vi "MainScript.vi"() -> ()   [LabVIEW 2020]
uses:
  <vilib>/Platform/TimedLoop/XDataNode/timing_clust.ctl
  <vilib>/Platform/TimedLoop/XDataNode/nitl_modes.ctl
  <vilib>/Platform/TimedLoop/XDataNode/wakeup.ctl
  Global 2.vi
  <vilib>/imath/engines/lvmath2/RunTimeEngine/Managers/WorkSpace/UID Generator.vi
  <vilib>/imath/engines/lvmath2/RunTimeEngine/RunTimeType/NIMS_RunTimeType_From StrictType (excl LVString).vi
  <instcachedir>/0/NIMS_RunTimeType_From StrictType (excl LVString)_283B1B2000484AAA8744D21CE97EA49F.lvgen/NIMS_RunTimeType_From StrictType (excl LVString)_283B1B2000484AAA8744D21CE97EA49F_000.vi
  <vilib>/imath/engines/lvmath2/RunTimeEngine/LocalVariableDefStatement/MC_LocalVariableDefStatement_Display.vi
  <vilib>/imath/engines/lvmath2/RunTimeEngine/Managers/SymbolTable/Clear UID.vi
  <vilib>/imath/engines/lvmath2/RunTimeEngine/NodeEndStatement/NIMS_NodeEndStatement_Output.vi
  <instcachedir>/0/NIMS_NodeEndStatement_Output_53EC0D466D134D7ABD903AC30B43404B.lvgen/NIMS_NodeEndStatement_Output_53EC0D466D134D7ABD903AC30B43404B_005.vi
  <vilib>/imath/engines/lvmath2/RunTimeEngine/ErrorHandling/NIMS_Finalize Error.vi
  <vilib>/Platform/TimedLoop/XDataNode/loadnilvce.vi
  <vilib>/imath/engines/lvmath2/RunTimeEngine/RangeToken/NIMS_Range_R2 - Integer.vi
  <instcachedir>/0/NIMS_Range_R2 - Integer_FFC1A4B1B9F04947ABCB56F009996D55.lvgen/NIMS_Range_R2 - Integer_FFC1A4B1B9F04947ABCB56F009996D55_000.vi
  <vilib>/imath/engines/lvmath2/RunTimeEngine/CommandStatement/MC_CommandStatement_break.vi
  <vilib>/imath/engines/lvmath2/RunTimeEngine/MatrixToken/NIMS_MatrixToken_M_SorCV.vi
  <instcachedir>/0/NIMS_MatrixToken_M_SorCV_D62667310BD447638EB690CBF8A818C2.lvgen/NIMS_MatrixToken_M_SorCV_D62667310BD447638EB690CBF8A818C2_000.vi
  <vilib>/imathl/engines/lvmath/Functions/Error Handling/Create Error.vi
  <vilib>/imath/engines/lvmath2/RunTimeEngine/IndexRead/NIMS M(S).vi
  <instcachedir>/0/NIMS M(S)_B826C018497E4940AE96BD27B540B6FB.lvgen/NIMS M(S)_B826C018497E4940AE96BD27B540B6FB_000.vi
  <vilib>/imath/engines/lvmath2/RunTimeEngine/MatrixToken/NIMS_MatrixToken_M_M.vi
  <instcachedir>/0/NIMS_MatrixToken_M_M_70A974A5272043BBA0045176BCC4D8A7.lvgen/NIMS_MatrixToken_M_M_70A974A5272043BBA0045176BCC4D8A7_004.vi
  <vilib>/imath/engines/lvmath2/RunTimeEngine/ErrorHandling/NIMS_Create Error From Enums.vi
  <vilib>/imath/engines/lvmath2/RunTimeEngine/BuiltInFunctions/length/NIMS_length(GV).vi
  <instcachedir>/0/NIMS_length(GV)_08A3D13377FD4E4B96F5795FBF3698FA.lvgen/NIMS_length(GV)_08A3D13377FD4E4B96F5795FBF3698FA_000.vi
  <vilib>/imath/engines/lvmath2/RunTimeEngine/BuiltInFunctions/zeros/NIMS_V=zeros(I32,I32).vi
  <vilib>/imath/engines/lvmath2/RunTimeEngine/RowToken/NIMS_RowToken_CV_CV.vi
  <instcachedir>/0/NIMS_RowToken_CV_CV_E2834F2F68C5494A92C49C498959A73E.lvgen/NIMS_RowToken_CV_CV_E2834F2F68C5494A92C49C498959A73E_000.vi
  <vilib>/imath/engines/lvmath2/RunTimeEngine/RowToken/NIMS_RowToken_M_CV.vi
  <instcachedir>/0/NIMS_RowToken_M_CV_79C297319A314039B767729C6880A213.lvgen/NIMS_RowToken_M_CV_79C297319A314039B767729C6880A213_000.vi
  <vilib>/imath/engines/lvmath2/RunTimeEngine/BuiltInFunctions/size/NIMS_[I32,I32]=size(GM).vi
  <instcachedir>/0/NIMS_[I32,I32]=size(GM)_B0A6EC1255BB4C8AB801FE6F734128D9.lvgen/NIMS_[I32,I32]=size(GM)_B0A6EC1255BB4C8AB801FE6F734128D9_000.vi
  <vilib>/imath/engines/lvmath2/RunTimeEngine/IndexRead/NIMS M($,S).vi
  <instcachedir>/0/NIMS M($,S)_3E5749BBB62E49528D4765A77F1F6D98.lvgen/NIMS M($,S)_3E5749BBB62E49528D4765A77F1F6D98_000.vi
  <vilib>/imath/engines/lvmath2/RunTimeEngine/ArithmeticOperatorToken/NIMS_ArithmeticOperator_plus.vi
  <instcachedir>/0/NIMS_ArithmeticOperator_plus_54468E2FAC2848C4BF0D457641184E60.lvgen/NIMS_ArithmeticOperator_plus_54468E2FAC2848C4BF0D457641184E60_004.vi
  <vilib>/imath/engines/lvmath2/RunTimeEngine/IndexRead/NIMS M(S,$).vi
  <instcachedir>/0/NIMS M(S,$)_F24F360562DE41D8BE234322A2E15C65.lvgen/NIMS M(S,$)_F24F360562DE41D8BE234322A2E15C65_000.vi
  <instcachedir>/0/NIMS_NodeEndStatement_Output_53EC0D466D134D7ABD903AC30B43404B.lvgen/NIMS_NodeEndStatement_Output_53EC0D466D134D7ABD903AC30B43404B_002.vi
  <vilib>/imath/engines/lvmath2/RunTimeEngine/IndexReplace/NIMS M(S,S)=S.vi
  <instcachedir>/0/NIMS M(S,S)=S_FBAB070788A64735BCFA47F7F92815DB.lvgen/NIMS M(S,S)=S_FBAB070788A64735BCFA47F7F92815DB_000.vi
  <instcachedir>/0/NIMS M(S,S)=S_FBAB070788A64735BCFA47F7F92815DB.lvgen/NIMS M(S,S)=S_FBAB070788A64735BCFA47F7F92815DB_002.vi
  <vilib>/imath/engines/lvmath2/RunTimeEngine/CommandStatement/NIMS_CommandStatement_MaskErr.vi
  <vilib>/imath/engines/lvmath2/RunTimeEngine/ArithmeticOperatorToken/NIMS_ArithmeticOperator_multmx-internal.vi
  <instcachedir>/0/NIMS_ArithmeticOperator_multmx-internal_B44B9A6937C8407A9A8862E3F2935EB3.lvgen/NIMS_ArithmeticOperator_multmx-internal_B44B9A6937C8407A9A8862E3F2935EB3_004.vi
  <vilib>/imath/engines/lvmath2/RunTimeEngine/BuiltInFunctions/length/NIMS_length(GM).vi
  <instcachedir>/0/NIMS_length(GM)_47CEC356FCE0482D9BA47DC61C99F2C7.lvgen/NIMS_length(GM)_47CEC356FCE0482D9BA47DC61C99F2C7_000.vi
  <instcachedir>/0/NIMS M(S)_B826C018497E4940AE96BD27B540B6FB.lvgen/NIMS M(S)_B826C018497E4940AE96BD27B540B6FB_005.vi
  <vilib>/imath/engines/lvmath2/RunTimeEngine/ArithmeticOperatorToken/NIMS_ArithmeticOperator_multmx(M,CV)-internal.vi
  <instcachedir>/0/NIMS_ArithmeticOperator_multmx(M,CV)-internal_19A14CC5BE0A4D31BE1E94A2E998D8C3.lvgen/NIMS_ArithmeticOperator_multmx(M,CV)-internal_19A14CC5BE0A4D31BE1E94A2E998D8C3_001.vi
  <vilib>/imath/engines/lvmath2/RunTimeEngine/IndexReplace/NIMS M($,S)=V.vi
  <instcachedir>/0/NIMS M($,S)=V_85A28EB895514E96A13A10261726EE3A.lvgen/NIMS M($,S)=V_85A28EB895514E96A13A10261726EE3A_001.vi
  <vilib>/imath/engines/lvmath2/RunTimeEngine/RowToken/NIMS_RowToken_M_M.vi
  <instcachedir>/0/NIMS_RowToken_M_M_23B851CD98934479877138710C79658F.lvgen/NIMS_RowToken_M_M_23B851CD98934479877138710C79658F_004.vi
  <vilib>/imath/engines/lvmath2/RunTimeEngine/IndexReplace/NIMS M(S)=S.vi
  <instcachedir>/0/NIMS M(S)=S_033E230F5F1E47BAA81748F03F1A64B6.lvgen/NIMS M(S)=S_033E230F5F1E47BAA81748F03F1A64B6_001.vi
  <vilib>/imath/engines/lvmath2/RunTimeEngine/NodeEndStatement/NIMS_NodeEndStatement_Get Vector.vi
  <instcachedir>/0/NIMS_NodeEndStatement_Get Vector_F9EEA26507564AFBA1E30D500A99934B.lvgen/NIMS_NodeEndStatement_Get Vector_F9EEA26507564AFBA1E30D500A99934B_001.vi
  <vilib>/imath/engines/lvmath/Functions/Error Handling/MergeErrorsWrapper.vi
  <instcachedir>/0/NIMS_NodeEndStatement_Output_53EC0D466D134D7ABD903AC30B43404B.lvgen/NIMS_NodeEndStatement_Output_53EC0D466D134D7ABD903AC30B43404B_009.vi
  <vilib>/imath/engines/lvmath2/RunTimeEngine/BuiltInFunctions/norm/NIMS_norm(GV,DBL).vi
  <instcachedir>/0/NIMS_norm(GV,DBL)_118B4CCB667A4D7498CD7C123070720C.lvgen/NIMS_norm(GV,DBL)_118B4CCB667A4D7498CD7C123070720C_000.vi
  <vilib>/imath/engines/lvmath2/RunTimeEngine/IndexRead/NIMS V(S).vi
  <instcachedir>/0/NIMS V(S)_0488751826AF41519A22953C041130DC.lvgen/NIMS V(S)_0488751826AF41519A22953C041130DC_000.vi
  <vilib>/imath/engines/lvmath2/RunTimeEngine/BuiltInFunctions/abs/NIMS_abs(signed).vi
  <instcachedir>/0/NIMS_abs(signed)_C4FCB8E6058B49B797C7C8D53CA5F6EC.lvgen/NIMS_abs(signed)_C4FCB8E6058B49B797C7C8D53CA5F6EC_000.vi
  <instcachedir>/0/NIMS_NodeEndStatement_Output_53EC0D466D134D7ABD903AC30B43404B.lvgen/NIMS_NodeEndStatement_Output_53EC0D466D134D7ABD903AC30B43404B_001.vi
  <vilib>/imath/engines/lvmath2/RunTimeEngine/BuiltInFunctions/cos/NIMS_cos(C).vi
  <instcachedir>/0/NIMS_cos(C)_9DC0D0878EF24EB8B280F2BED1FF8FCD.lvgen/NIMS_cos(C)_9DC0D0878EF24EB8B280F2BED1FF8FCD_001.vi
  <vilib>/imath/engines/lvmath2/RunTimeEngine/BuiltInFunctions/acos/NIMS_acos(C).vi
  <instcachedir>/0/NIMS_acos(C)_5BB0E87CCFB0408A9DC8B350AC83525E.lvgen/NIMS_acos(C)_5BB0E87CCFB0408A9DC8B350AC83525E_001.vi
  <instcachedir>/0/NIMS_RunTimeType_From StrictType (excl LVString)_283B1B2000484AAA8744D21CE97EA49F.lvgen/NIMS_RunTimeType_From StrictType (excl LVString)_283B1B2000484AAA8744D21CE97EA49F_009.vi
  <instcachedir>/0/NIMS_abs(signed)_C4FCB8E6058B49B797C7C8D53CA5F6EC.lvgen/NIMS_abs(signed)_C4FCB8E6058B49B797C7C8D53CA5F6EC_002.vi
  <vilib>/imath/engines/lvmath2/RunTimeEngine/RunTimeType/NIMS_RunTimeType_Set Source Original Bool.vi
  <instcachedir>/0/NIMS_NodeEndStatement_Output_53EC0D466D134D7ABD903AC30B43404B.lvgen/NIMS_NodeEndStatement_Output_53EC0D466D134D7ABD903AC30B43404B_010.vi
  <vilib>/platform/TimedLoop/XDataNode/XDataNode.xnode
  <vilib>/Platform/TimedLoop/XDataNode/XDNodeRunTimeDep.lvlib
  <vilib>/imath/engines/lvmath2/RunTimeEngine/Managers/SymbolTable/NIMS_WorkSpace.lvlib
panel:
  out "v2":dbl(graph)=-75141.23523042882
  out "v1":dbl(graph)=57052.989399066195
  out "Boolean":bool
  in  "CDB":dbl=-0.002
  in  "ThrustCoefB":dbl=0.00015
  in  "KdB":dbl
  in  "KiB":dbl
  in  "KpB":dbl=5.0
  in  "Reverse":bool
  out "Array":dbl[](array[numeric])=[-97.53326262976505, 22.07402728985534, 0.0]
  in  "CD":dbl=-0.002
  in  "Radio Buttons":enum32{"Racetrack", "Circular", "Tube"}(radio)=enum."Circular"
  in  "Racetrack length [mm]":dbl=60.0
  in  "Ractrack width [mm]":dbl=15.0
  out "Rotation speed [Hz]":dbl(graph)=50.0
  in  "Zscale":dbl=0.95
  in  "YScale":dbl=0.9
  in  "XScale":dbl=0.95
  in  "Zoffset":dbl=-0.073
  in  "Yoffset":dbl=-0.076
  in  "Xoffset":dbl=0.07
  out "?":bool
  in  "Centripedal force compensation":bool
  in  "KCentripedal force":dbl=0.007
  in  "?":bool=TRUE
  in  "Rot [Hz]":dbl=50.0
  in  "Rotational speed":bool
  in  "Traj_Rotate":bool
  in  "Omega_Max_change":dbl=20.0
  in  "Thrust coefficient [N.s/rad]":dbl=0.0002
  out "T4":dbl=29.408844544558946
  out "T1":dbl=27.525528387426544
  out "T2":dbl=30.561149827671912
  out "T3":dbl=31.865396803696214
  out "T5":dbl=28.858824483224712
  out "T6":dbl=28.760553201657874
  out "Z-":dbl(slide)=27.525528387426544 scale=0.0..100.0
  out "Z+":dbl(slide)=30.561149827671912 scale=0.0..100.0
  out "X-":dbl(slide)=31.865396803696214 scale=0.0..100.0
  out "X+":dbl(slide)=29.408844544558946 scale=0.0..100.0
  out "Y-":dbl(slide)=28.858824483224712 scale=0.0..100.0
  out "Y+":dbl(slide)=28.760553201657874 scale=0.0..100.0
  out "OverTemp":bool
  in  "Max Temp[C]":dbl=75.0
  in  "On Off":bool
  in  "Max Orientation change rate [rad/s]":dbl=15.0
  out "On":bool
  in  "Reset Integral":bool
  in  "Force Vertical":bool
  in  "Robot Mass [Kg]":dbl=5e-05
  in  "Kd":dbl
  in  "Ki":dbl=1e-05
  in  "Kp":dbl=0.5
  out "XZ View":T1(graph)=[{"XCircleBot"=[0.0114245818886292, 0.011179747012409945, 0.010505186500365478, 0.009566056291964605, 0.008592288215534915, 0.007822294657535332, 0.007444596895428308, 0.007551668514047607, 0.008117294646901975, 0.00900299028976764, 0.009991906259555651, 0.010841921437211719, 0.011344922461929932], "YCircleBot"=[-0.07472721060762046, -0.07376835953041205, -0.07304426863800466, -0.07273222063441234, -0.07290861575396909, -0.07353026631941255, -0.07444497059150072, -0.07542877706299969, -0.07624081559823631, -0.07668227084295065, -0.07664505915694673, -0.07613829125876125, -0.0752860416040183]}, {"XCircleBot"=array[1002 elements], "YCircleBot"=array[1002 elements]}, {"XCircleBot"=[0.008713695894261728, 0.008468861018042473, 0.007794300505998007, 0.006855170297597133, 0.005881402221167443, 0.0051114086631678605, 0.0047337109010608365, 0.004840782519680135, 0.0054064086525345036, 0.0062921042954001685, 0.0072810202651881805, 0.008131035442844247, 0.008634036467562459], "YCircleBot"=[0.0, 0.000958851077208406, 0.0016829419696157931, 0.001994989973208109, 0.0018185948536513636, 0.0011969442882079132, 0.0002822400161197344, -0.0007015664553792397, -0.0015136049906158565, -0.001955060235330194, -0.001917848549326277, -0.001411080651140784, -0.0005588309963978518]}, {"XCircleBot"=[0.0094245818886292, 0.012626616728347043], "YCircleBot"=[-0.07472721060762046, -0.02564219522787055]}]
  out "XY View":T1(graph)=[{"XCircleBot"=[0.0114245818886292, 0.011179747012409945, 0.010505186500365478, 0.009566056291964605, 0.008592288215534915, 0.007822294657535332, 0.007444596895428308, 0.007551668514047607, 0.008117294646901975, 0.00900299028976764, 0.009991906259555651, 0.010841921437211719, 0.011344922461929932], "YCircleBot"=[0.041338273099899805, 0.04229712417710821, 0.043021215069515596, 0.04333326307310791, 0.04315686795355117, 0.04253521738810772, 0.04162051311601954, 0.040636706644520564, 0.03982466810928395, 0.03938321286456961, 0.03942042455057353, 0.03992719244875902, 0.040779442103501956]}, {"XCircleBot"=array[1002 elements], "YCircleBot"=array[1002 elements]}, {"XCircleBot"=[0.008713695894261728, 0.008468861018042473, 0.007794300505998007, 0.006855170297597133, 0.005881402221167443, 0.0051114086631678605, 0.0047337109010608365, 0.004840782519680135, 0.0054064086525345036, 0.0062921042954001685, 0.0072810202651881805, 0.008131035442844247, 0.008634036467562459], "YCircleBot"=[0.029239122486290382, 0.03019797356349879, 0.030922064455906176, 0.031234112459498493, 0.031057717339941747, 0.030436066774498297, 0.029521362502410116, 0.028537556030911144, 0.027725517495674527, 0.027284062250960188, 0.027321273936964104, 0.0278280418351496, 0.02868029148989253]}, {"XCircleBot"=[0.0094245818886292, 0.012626616728347043], "YCircleBot"=[0.041338273099899805, 0.03237120902881452]}]
  out "Loop Duration [ms]":u32(graph)=3
  out "Max Current [A]":dbl(knob)=3.0 scale=0.0..2.0
  out "Current Saturation":bool=TRUE
  in  "Max Current [A]":dbl=3.0
  in  "Flux density magnitude (mT)":dbl=3.0
  in  "stop":bool
  # "Program performance monitoring"
  # "Program control"
  # "User Input"
  # "Auto"
  # "Manual"
  # "Show Direction Setpoint"
  # "Current control mode"
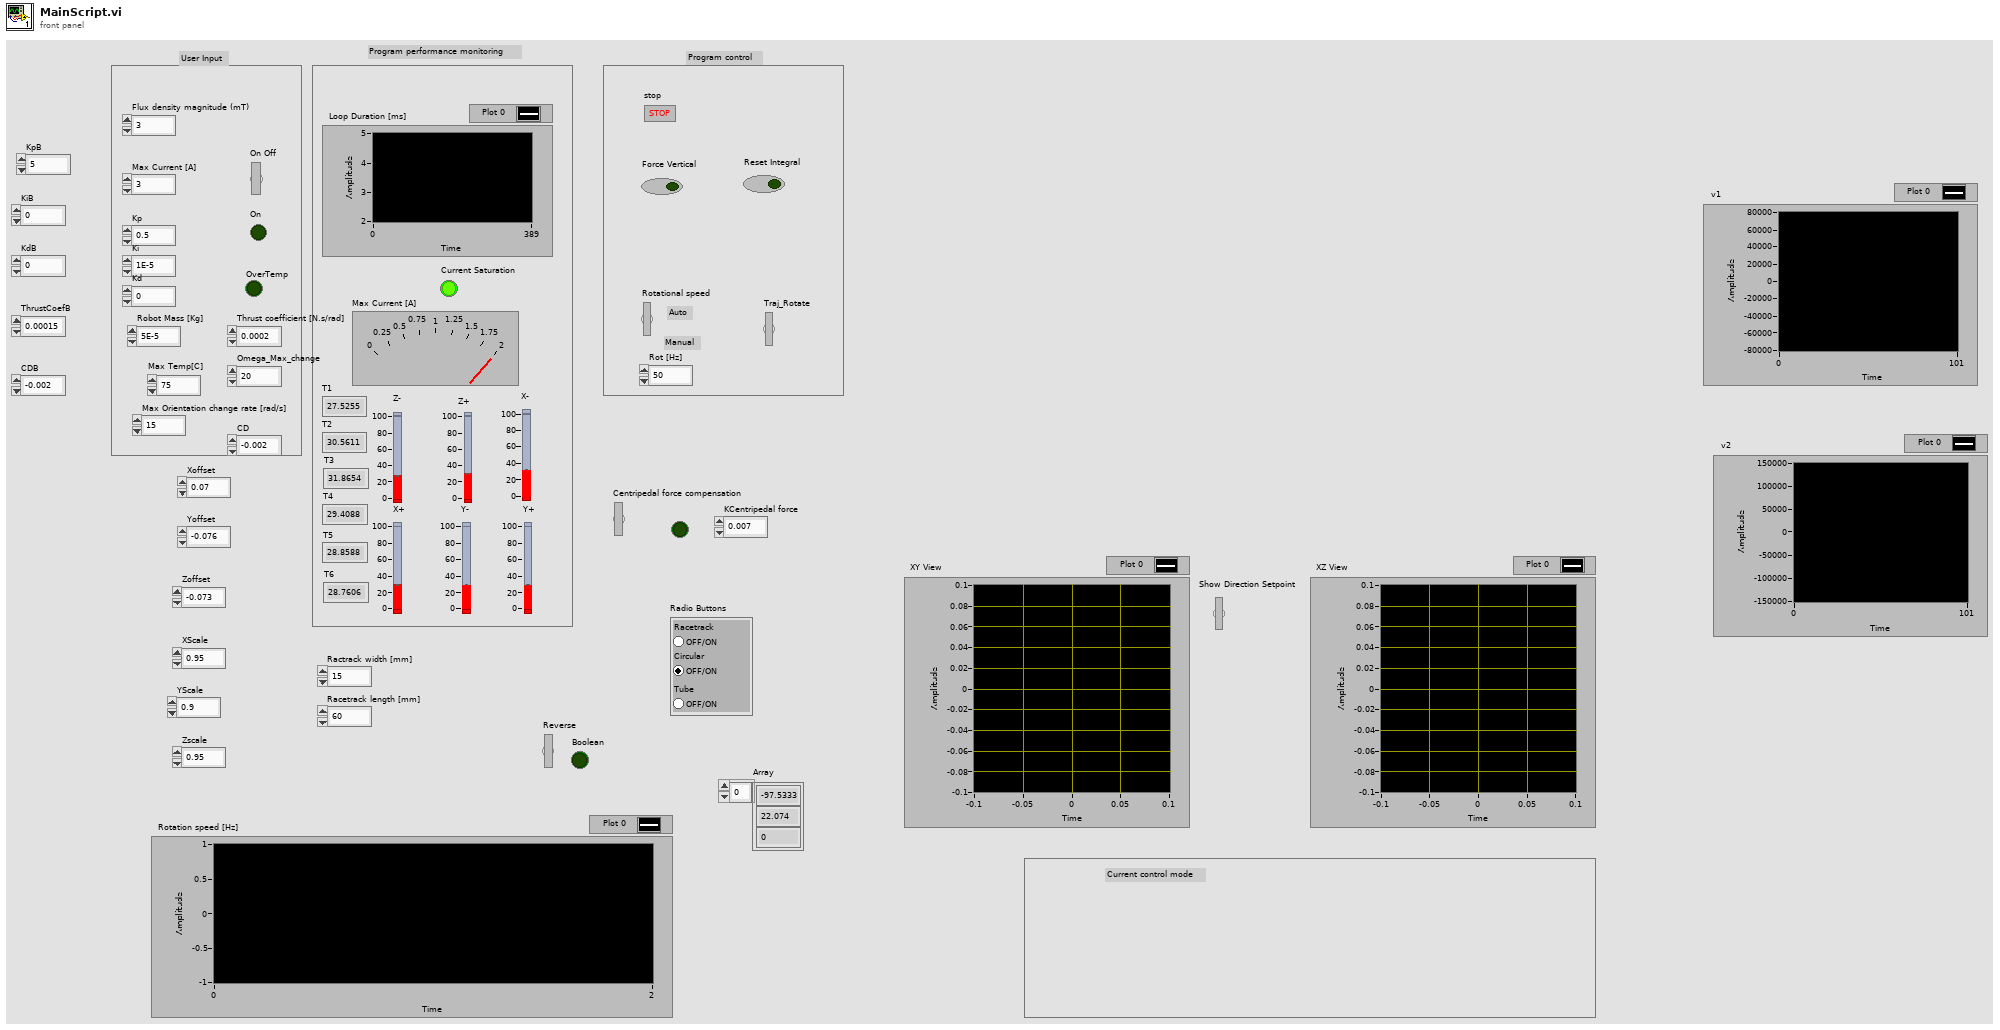
[diagram p1: front panel]
types:
  T1 = cluster{"XCircleBot":dbl[], "YCircleBot":dbl[]}[]
  T2 = typedef "XDNodeRunTimeDep.lvlib/timing_clust.ctl" = cluster{"Expected End [f-1]":u64, "Actual End [f-1]":u64, "Finished Late? [f-1]":bool, "Expected End [i-1]":u64, "Actual End [i-1]":u64, "Finished Late? [i-1]":bool, "Expected Start [i]":u64, "Actual Start [i]":u64, "Expected Start [f]":u64, "Actual Start [f]":u64, "Source Name":string, "Structure Name":string, "Period":i64, "Deadline":i64, "Offset":i64, "Start":i64, "Priority":i32, "Timeout":i32, "Mode":T3, "Wakeup Reason":T4, "Error":errorcluster, "Source Type":string, "Secondary Source Type":string, "Global End Time":u64, "Global Start Time":u64, "Frame Duration":u64, "Iteration Duration":u64, "Assigned CPU":i32, "I/O Scan Engine Mode":u32}
  T3 = typedef "XDNodeRunTimeDep.lvlib/nitl_modes.ctl" = enum32{"No Change", "Process missed periods, maintain original phase", "Discard missed periods, maintain original phase", "Process missed periods, ignore original phase", "Discard missed periods, ignore original phase"}
  T4 = typedef "XDNodeRunTimeDep.lvlib/wakeup.ctl" = enum32{"Normal", "Aborted", "Asynchronous wakeup", "Timing source error", "Timed loop error", "Timeout"}
  T5 = cluster{"XCircleClosestOut":dbl[], "ZCircleClosestOut":dbl[]}
  T6 = cluster{"XCircleBotOut":dbl[], "ZCircleBotOut":dbl[]}
  T7 = cluster{"XCircleClosestOut":dbl[], "YCircleClosestOut":dbl[]}
  T8 = cluster{"XCircleBotOut":dbl[], "YCircleBotOut":dbl[]}
  T9 = cluster{cluster{"XCircleBotOut":dbl[], "ZCircleBotOut":dbl[]}, cluster{"XHD":dbl[], "ZHD":dbl[]}, cluster{"XCircleClosestOut":dbl[], "ZCircleClosestOut":dbl[]}, cluster{"XPlot":dbl[], "ZPlot":dbl[]}}
  T10 = cluster{cluster{"XCircleBotOut":dbl[], "YCircleBotOut":dbl[]}, cluster{"XHD":dbl[], "YHD":dbl[]}, cluster{"XCircleClosestOut":dbl[], "YCircleClosestOut":dbl[]}, cluster{"XPlot":dbl[], "YPlot":dbl[]}}
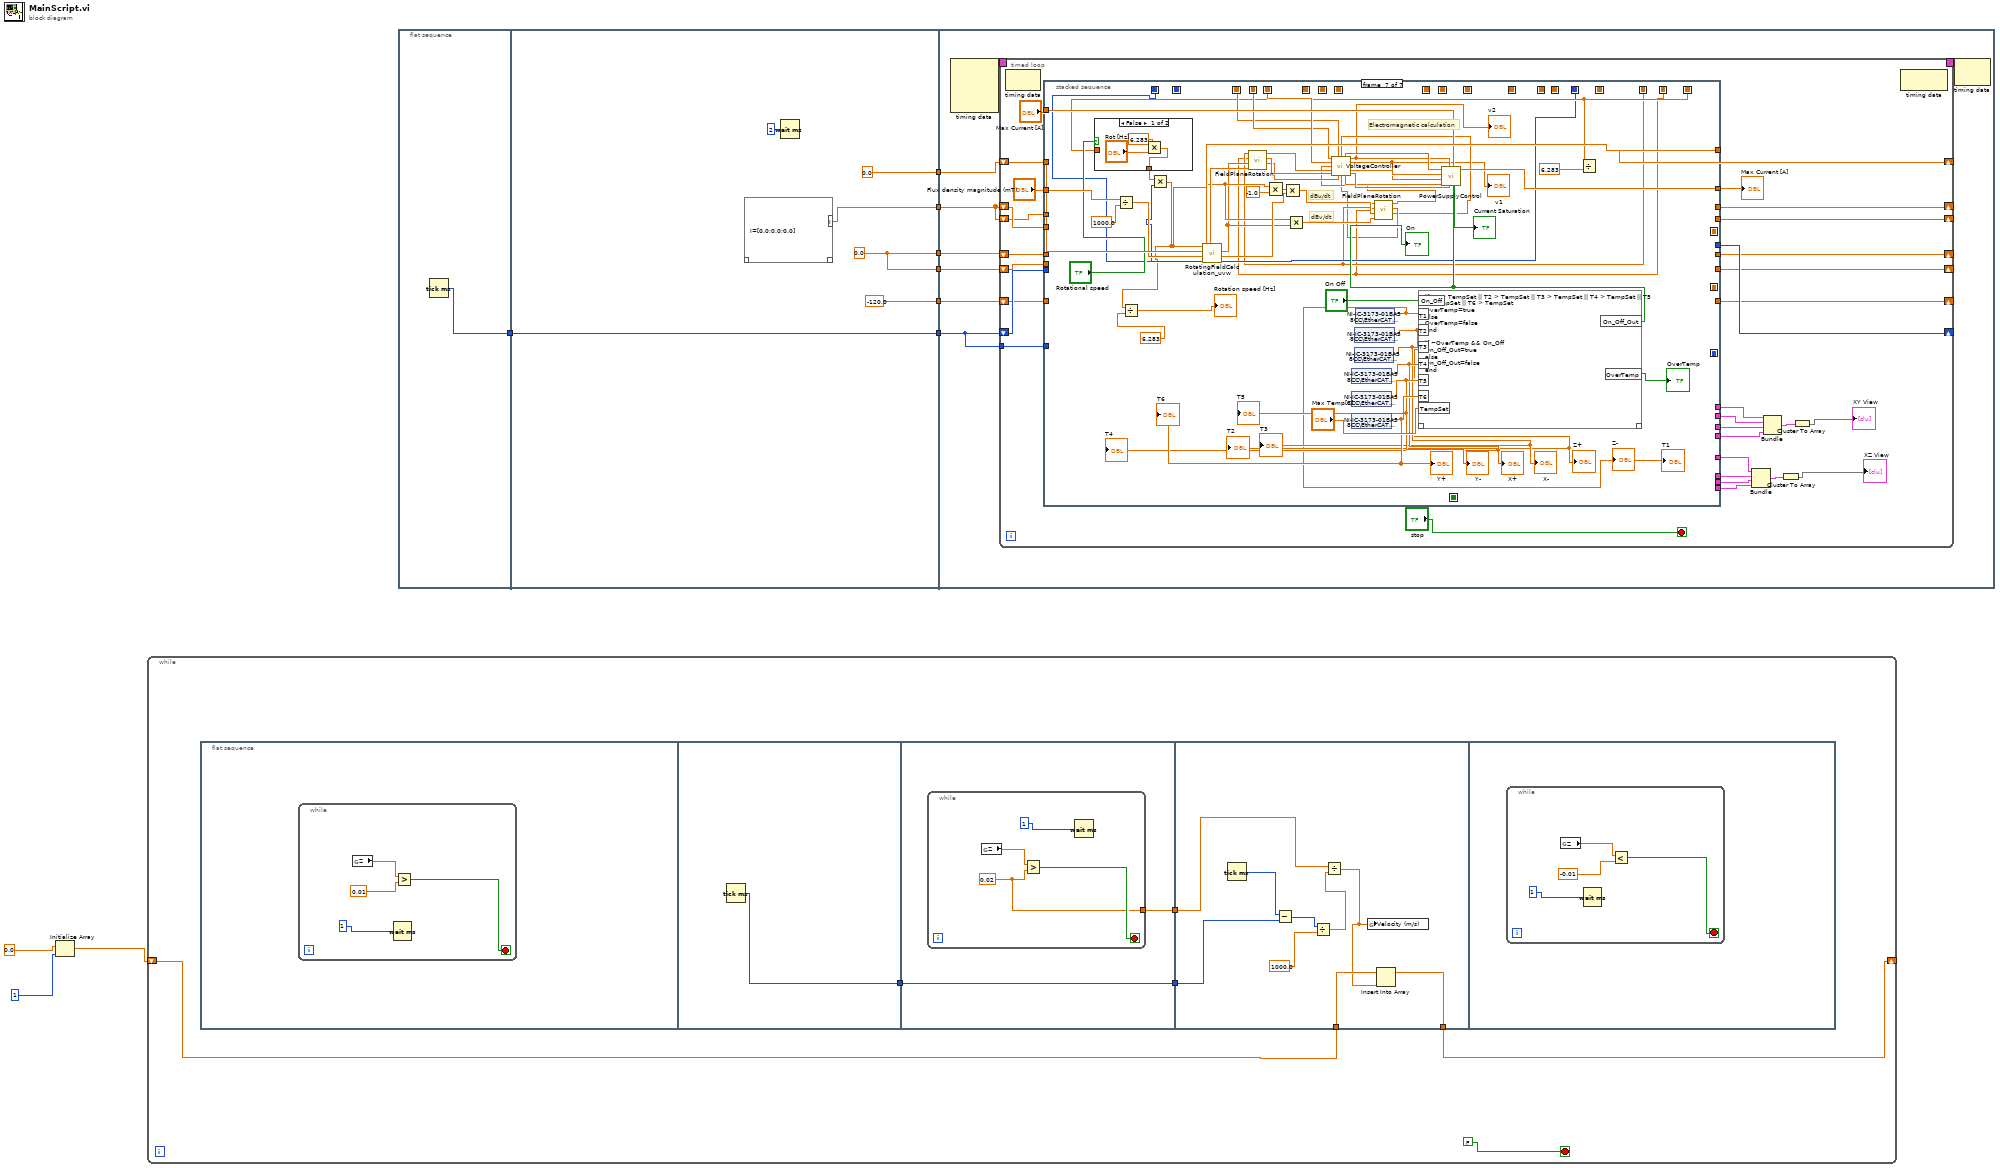
[diagram p0: block diagram]
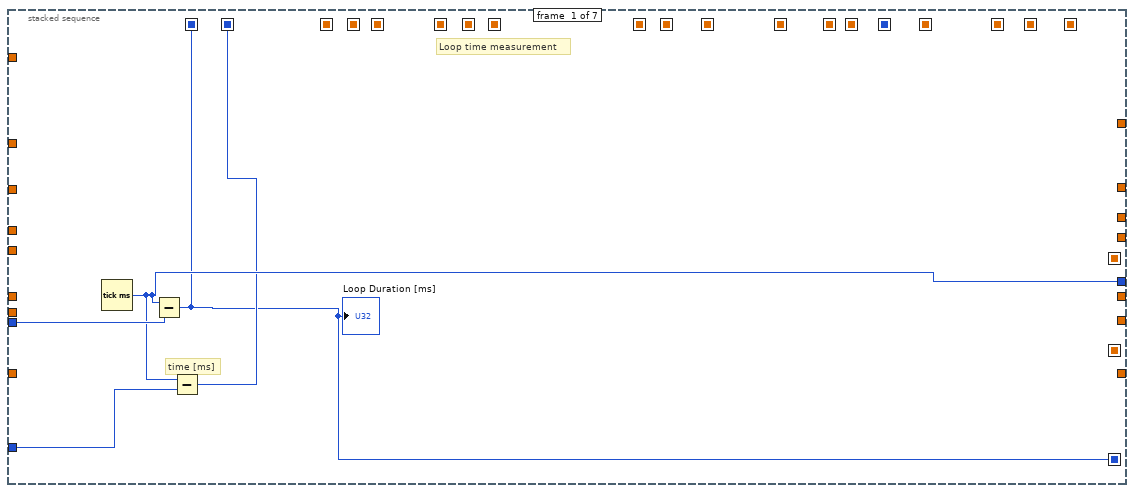
[diagram p2: hidden frame]
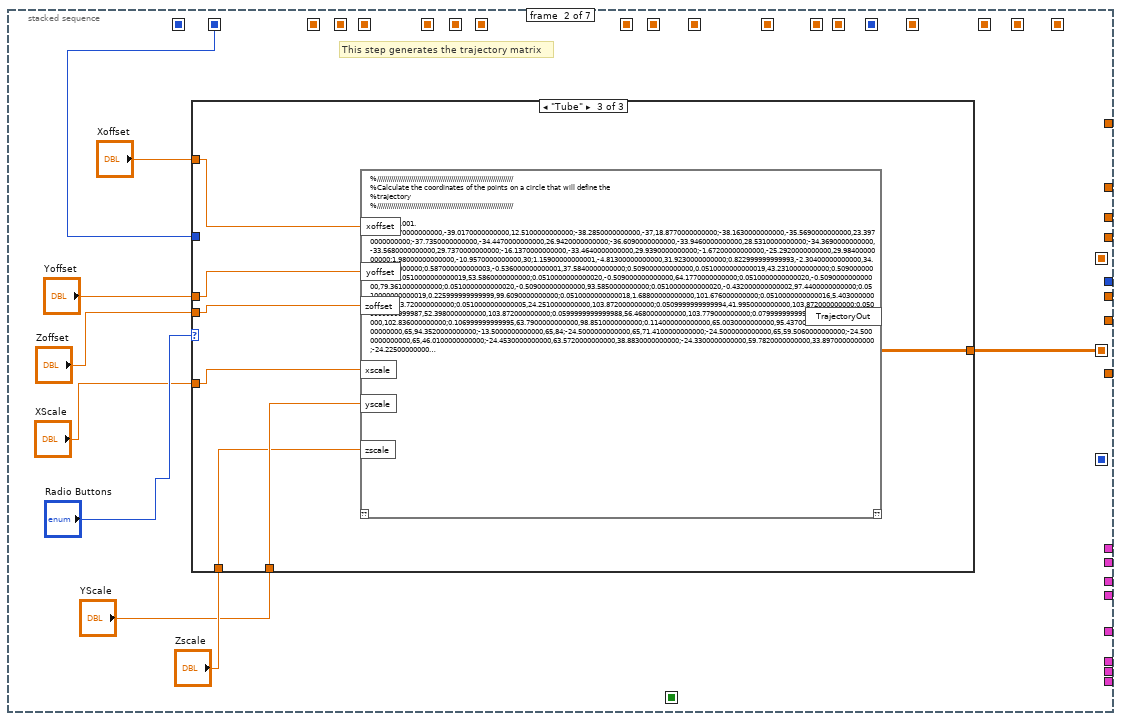
[diagram p3: hidden frame]
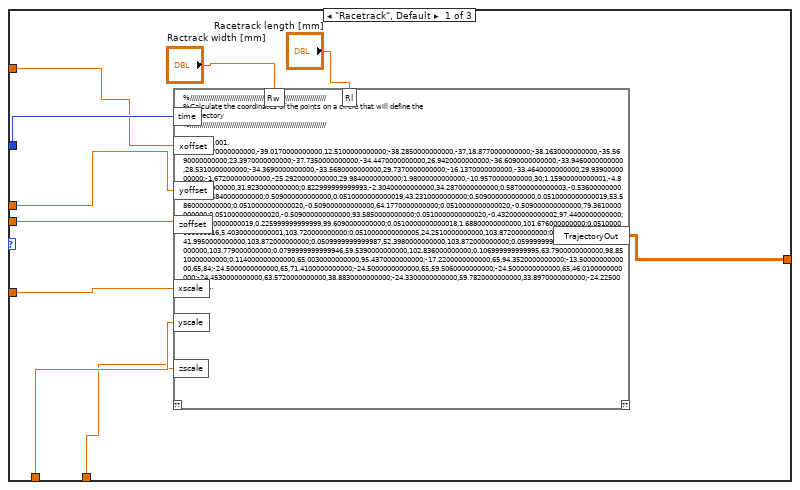
[diagram p4: hidden frame]
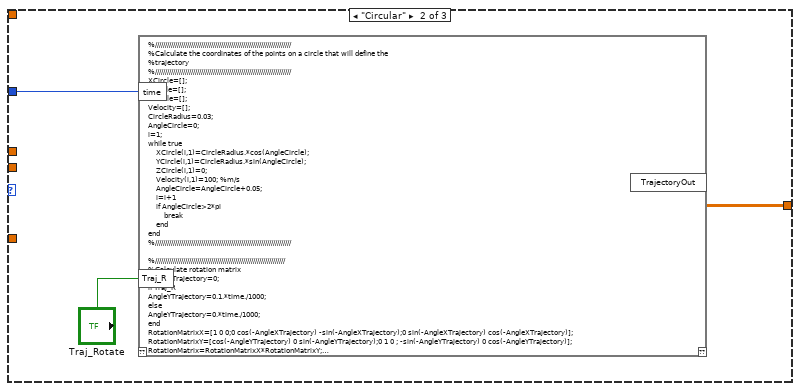
[diagram p5: hidden frame]
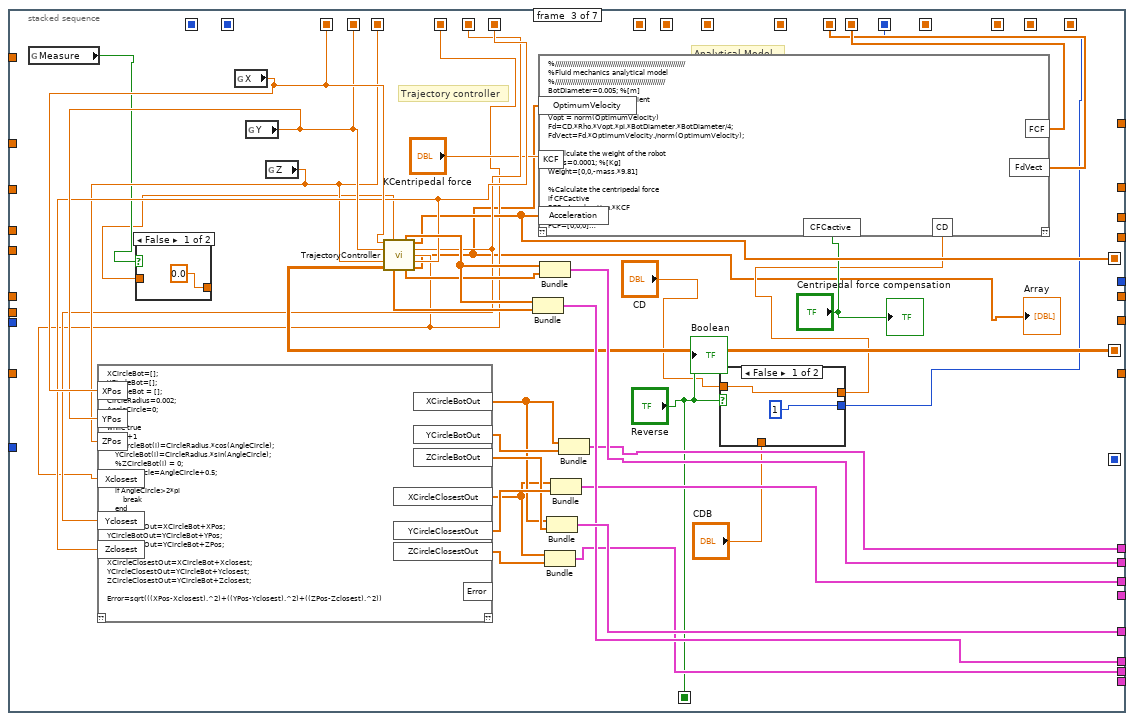
[diagram p6: hidden frame]
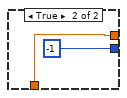
[diagram p7: hidden frame]
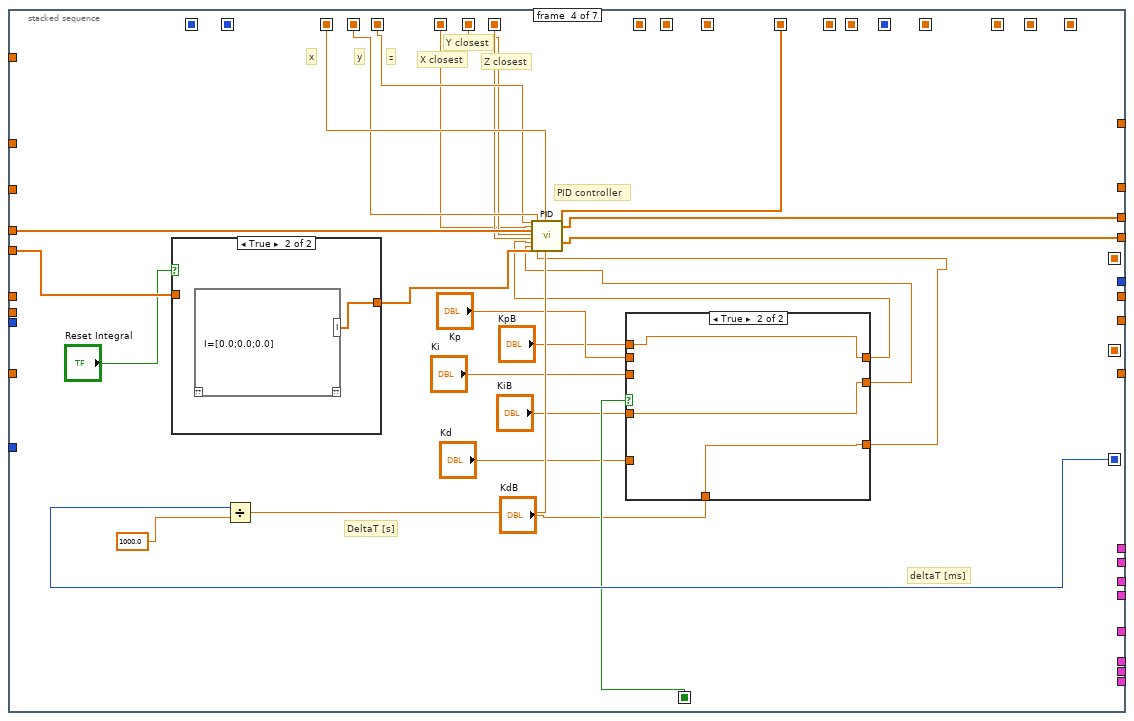
[diagram p9: hidden frame]
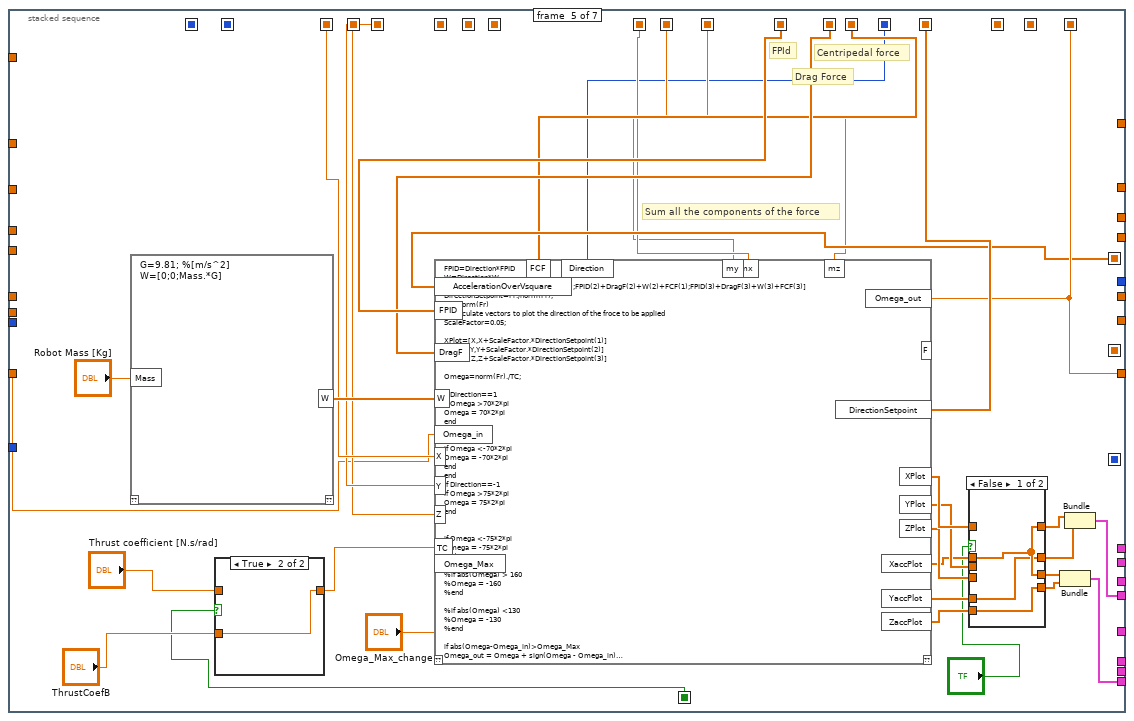
[diagram p12: hidden frame]
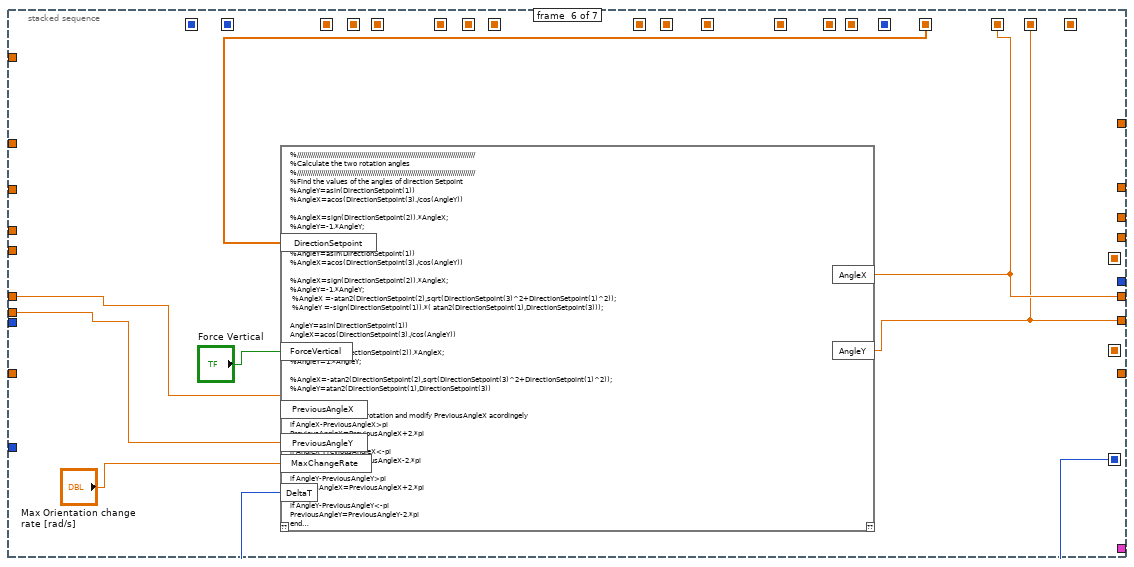
[diagram p15: hidden frame]
diagram:
  n1 = Initialize Array(0.0, 1) -> (w3:dbl[])
  n2 = while {
    shift-right: [w11] -> _
    shift-left: w3 -> [w12]
    stop <- FALSE stop-if-true
    n3 = flat-sequence {
      tunnel: [w21] -> w15
      tunnel: w15 -> [w23]
      tunnel: [w23] -> w14
      tunnel: [w22] -> w13
      tunnel: w14 -> [w35]
      tunnel: w13 -> [w34]
      tunnel: [w31] -> w11
      tunnel: w12 -> [w30]
      frame #0 {
        n4 = while {
          stop <- w18 stop-if-true
          n5 = global read "Global 2.vi" "Z"() -> (w20:dbl)
          n6 = Wait (ms)(milliseconds to wait=1) -> ()  [unwired: 1 out]
          n7 = Greater?(x=w20, y=0.01) -> (0:w18:bool)
        }
      }
      frame #1 {
        n8 = Tick Count (ms)() -> (millisecond timer value=w21:u32)
      }
      frame #2 {
        n9 = while {
          tunnel: [w24] -> w22
          stop <- w26 stop-if-true
          w24 = 0.02
          n10 = global read "Global 2.vi" "Z"() -> (w27:dbl)
          n11 = Greater?(x=w27, y=w24) -> (0:w26:bool)
          n12 = Wait (ms)(milliseconds to wait=1) -> ()  [unwired: 1 out]
        }
      }
      frame #3 {
        n13 = Tick Count (ms)() -> (millisecond timer value=w36:u32)
        n14 = Subtract(x=w36, y=w35) -> (x-y=w33:u32)
        n15 = Divide(x=w33, y=1000.0) -> (x/y=w29:dbl)
        n16 = Divide(x=w34, y=w29) -> (x/y=w28:dbl)
        n17 = global write "Global 2.vi" "Velocity (m/s)"(w28) -> ()
        n18 = Insert Into Array(array=w30, new element=w28) -> (w31:dbl[])  [unwired: 1 in]
      }
      frame #4 {
        n19 = while {
          stop <- w38 stop-if-true
          n20 = global read "Global 2.vi" "Z"() -> (w40:dbl)
          n21 = Wait (ms)(milliseconds to wait=1) -> ()  [unwired: 1 out]
          n22 = Less?(x=w40, y=-0.01) -> (x < y?=w38:bool)
        }
      }
    }
  }
  n23 = flat-sequence {
    tunnel: [w41] -> w8
    tunnel: [w46] -> w10
    tunnel: [0.0] -> w9
    tunnel: w8 -> [w46]
    tunnel: [w44] -> w7
    tunnel: [w43] -> w6
    tunnel: [w43] -> w5
    tunnel: [-120.0] -> w4
    tunnel: w10 -> [w81]
    tunnel: w9 -> [w85]
    tunnel: w7 -> [w84]
    tunnel: w6 -> [w83]
    tunnel: w5 -> [w82]
    tunnel: w4 -> [w80]
    frame #0 {
      n24 = Tick Count (ms)() -> (millisecond timer value=w41:u32)
    }
    frame #1 {
      w43 = 0.0
      n25 = mathscript code="I=[0.0;0.0;0.0]"() -> ("I"=w44:dbl[])  [unwired: 1 in, 1 out]
      n26 = Wait (ms)(milliseconds to wait=u32 2) -> ()  [unwired: 1 out]
    }
    frame #2 {
      n27 = node-c288() -> (w87:T2)  [unwired: 4 in]
      n28 = timed-loop {
        timing: w87 -> [_]
        timing-out: [_] -> w86
        shift-right: [w111] -> _
        shift-left: w81 -> [w112]
        shift-right: [w117] -> _
        shift-left: w85 -> [w116]
        shift-right: [w110] -> _
        shift-left: w84 -> [w109]
        shift-right: [w108] -> _
        shift-left: w84 -> [w107]
        shift-right: [w106] -> _
        shift-left: w83 -> [w104]
        shift-right: [w105] -> _
        shift-left: w82 -> [w103]
        tunnel: w81 -> [w90]
        shift-right: [w89] -> _
        shift-left: w80 -> [w88]
        stop <- "stop" stop-if-true
        n29 = node-c288() -> ()  [unwired: 1 in, 1 out]
        n30 = stacked-sequence {
          seq-local: [_ w131 _ _ _ _ _] -> [_ _ w1456 _ _ _ _]
          seq-local: [w119 _ _ _ _ _ _] -> [_ _ _ w1985 _ w2895 _]
          seq-local: [_ _ w1458 _ _ _ _] -> [_ _ _ w1991 w2063 _ w3315]
          seq-local: [_ _ w1457 _ _ _ _] -> [_ _ _ w1990 w2062 _ w3316]
          seq-local: [_ _ w1451 _ _ _ _] -> [_ _ _ w1989 w2061 _ w3317]
          seq-local: [_ _ w1445 _ _ _ _] -> [_ _ _ w1986 _ _ _]
          seq-local: [_ _ w1450 _ _ _ _] -> [_ _ _ w1987 _ _ _]
          seq-local: [_ _ w1452 _ _ _ _] -> [_ _ _ w1988 _ _ _]
          seq-local: [_ _ _ w1982 _ _ _] -> [_ _ _ _ w2066 _ _]
          seq-local: [_ _ w1442 _ _ _ _] -> [_ _ _ _ w2065 _ _]
          seq-local: [_ _ _ _ w2064 _ _] -> [_ _ _ _ _ w2897 _]
          seq-local: [_ _ _ _ _ w2891 _] -> [_ _ _ _ _ _ w3299]
          seq-local: [_ _ _ _ _ w2890 _] -> [_ _ _ _ _ _ w3298]
          seq-local: [w120 _ _ _ _ _ _] -> [_ w132 _ _ _ _ _]
          seq-local: [_ _ _ _ w2058 _ _] -> [_ _ _ _ _ _ w3312]
          seq-local: [w119 _ _ _ _ _ _] -> [_ _ _ _ _ _ w3311]
          seq-local: [_ _ w1449 _ _ _ _] -> [_ _ _ _ w2055 _ _]
          seq-local: [_ _ w1447 _ _ _ _] -> [_ _ _ _ w2043 _ _]
          seq-local: [_ _ _ _ w2042 _ _] -> [_ _ _ _ _ _ _]
          seq-local: [_ _ _ _ w2041 _ _] -> [_ _ _ _ _ _ _]
          seq-local: [_ _ _ _ w2040 _ _] -> [_ _ _ _ _ _ _]
          seq-local: [_ _ w1441 _ _ _ _] -> [_ _ _ _ w2039 _ w3307]
          seq-local: [_ _ "Reverse" _ _ _ _] -> [_ _ _ w1978 w2035 _ _]
          tunnel: [_ _ _ _ _ _ w3342] -> w117
          tunnel: w116 -> [_ _ _ _ _ _ w3341]
          tunnel: "Flux density magnitude (mT)" -> [_ _ _ _ _ _ w3330]
          tunnel: [_ _ _ _ _ _ w3329] -> w114
          tunnel: "Max Current [A]" -> [_ _ _ _ _ _ w3328]
          tunnel: w112 -> [w123 _ _ _ _ _ _]
          tunnel: [w122 _ _ _ _ _ _] -> w111
          tunnel: [_ _ _ w1994 _ _ _] -> w110
          tunnel: w109 -> [_ _ _ w1981 _ _ _]
          tunnel: [_ _ _ w1993 _ _ _] -> w108
          tunnel: w107 -> [_ _ _ w1992 _ _ _]
          tunnel: [_ _ _ _ _ w2891 _] -> w106
          tunnel: [_ _ _ _ _ w2890 _] -> w105
          tunnel: w104 -> [_ _ _ _ _ w2893 _]
          tunnel: w103 -> [_ _ _ _ _ w2892 _]
          tunnel: [_ _ w1464 _ _ _ _] -> w100
          tunnel: [_ _ w1463 _ _ _ _] -> w99
          tunnel: [_ _ w1462 _ _ _ _] -> w98
          tunnel: [_ _ w1461 _ _ _ _] -> w95
          tunnel: [_ _ w1460 _ _ _ _] -> w94
          tunnel: [_ _ w1459 _ _ _ _] -> w93
          tunnel: [_ _ _ _ w2060 _ _] -> w92
          tunnel: [_ _ _ _ w2059 _ _] -> w91
          tunnel: w90 -> [w121 _ _ _ _ _ _]
          tunnel: [_ _ _ _ w2058 _ _] -> w89
          tunnel: w88 -> [_ _ _ _ w2057 _ _]
          frame #0 {
            # "time [ms]"
            # "Loop time measurement"
            n31 = Tick Count (ms)() -> (millisecond timer value=w122:u32)
            n32 = Subtract(x=w122, y=w123) -> (x-y=w119:u32)
            "Loop Duration [ms]" <- w119
            n33 = Subtract(x=w122, y=w121) -> (x-y=w120:u32)
          }
          frame #1 {
            # "This step generates the trajectory matrix"
            n34 = case shown="\"Tube\"" "Radio Buttons" {
              tunnel: [w141 w666 w1174] -> w131
              tunnel: w132 -> [w142 w668 _]
              tunnel: "XScale" -> [w138 _ w1170]
              tunnel: "Zoffset" -> [w137 _ w1171]
              tunnel: "Yoffset" -> [w136 _ w1173]
              tunnel: "Xoffset" -> [w135 _ w1172]
              tunnel: "Zscale" -> [w134 _ w1168]
              tunnel: "YScale" -> [w133 _ w1169]
              frame "Racetrack", Default {
                n35 = mathscript code="%////////////////////////////////////////////////////////////////////\n%Calculate the coordinates of the points on a circle that will define the\n%trajectory\n%////////////////////////////////////////////////////////////////////\n\n%Traj=0.001.*[-38.4570000000000,-39.0170000000000,12.5100000000000;-38.2850000000000,-37,18.8770000000000;-38.1630000000000,-35.5690000000000,23.3970000000000;-37.7350000000000,-34.4470000000000,26.9420000000000;-36.6090000000000,-33.9460000000000,28.5310000000000;-34.3690000000000,-33.5680000000000,29.7370000000000;-16.1370000000000,-33.4640000000000,29.9390000000000;-1.67200000000000,-25.2920000000000,29.9840000000000;1.98000000000000,-10.9570000000000,30;1.15900000000001,-4.81300000000000,31.9230000000000;0.822999999999993,-2.30400000000000,34.2870000000000;0.587000000000003,-0.536000000000001,37.5840000000000;0.509000000000000,0.0510000000000019,43.2310000000000;0.509000000000000,0.0510000000000019,53.5860000000000;0.0510000000000020,-0.509000000000000,64.1770000000000;0.0510000000000020,-0.509000000000000,79.3610000000000;0.0510000000000020,-0.509000000000000,93.5850000000000;0.0510000000000020,-0.432000000000002,97.4400000000000;0.0510000000000019,0.225999999999999,99.6090000000000;0.0510000000000018,1.68800000000000,101.676000000000;0.0510000000000016,5.40300000000001,103.720000000000;0.0510000000000005,24.2510000000000,103.872000000000;0.0509999999999994,41.9950000000000,103.872000000000;0.0509999999999987,52.3980000000000,103.872000000000;0.0599999999999988,56.4680000000000,103.779000000000;0.0799999999999946,59.5390000000000,102.836000000000;0.106999999999995,63.7900000000000,98.8510000000000;0.114000000000000,65.0030000000000,95.4370000000000;-17.2200000000000,65,94.3520000000000;-13.5000000000000,65,84;-24.5000000000000,65,71.4100000000000;-24.5000000000000,65,59.5060000000000;-24.5000000000000,65,46.0100000000000;-24.4530000000000,63.5720000000000,38.8830000000000;-24.3300000000000,59.7820000000000,33.8970000000000;-24.2250000000000,56.5810000000000,31.7900000000000;-24.1290000000000,53.6370000000000,30.7170000000000;-24.1060000000000,50.4100000000000,30.1660000000000;-24.7430000000000,47.2760000000000,29.3580000000000;-26.0920000000000,44.7010000000000,27.7300000000000;-29.3070000000000,42.4960000000000,23.9310000000000;-36.7150000000000,39.4140000000000,15.2170000000000;-39.0170000000000,38.4570000000000,12.5100000000000]\n%Traj=0.001.*[-38.4570000000000,-39.0170000000000,12.5100000000000;-38.2850000000000,-37,18.8770000000000;-38.1630000000000,-35.5690000000000,23.3970000000000;-37.7350000000000,-34.4470000000000,26.9420000000000;-36.6090000000000,-33.9460000000000,28.5310000000000;-34.3690000000000,-33.5680000000000,29.7370000000000;-16.1370000000000,-33.4640000000000,29.9390000000000;-1.67200000000000,-25.2920000000000,29.9840000000000;1.98000000000000,-10.9570000000000,30;1.15900000000001,-4.81300000000000,31.9230000000000;0.822999999999993,-2.30400000000000,34.2870000000000;0.587000000000003,-0.536000000000001,37.5840000000000;0.509000000000000,0.0510000000000019,43.2310000000000;0.509000000000000,0.0510000000000019,53.5860000000000;0.0510000000000020,-0.509000000000000,64.1770000000000;0.0510000000000020,-0.509000000000000,79.3610000000000;0.0510000000000020,-0.509000000000000,93.5850000000000;0.0510000000000020,-0.432000000000002,97.4400000000000;0.0510000000000019,0.225999999999999,99.6090000000000;0.0510000000000018,1.68800000000000,101.676000000000;0.0510000000000016,5.40300000000001,103.720000000000;0.0510000000000005,24.2510000000000,103.872000000000;0.0509999999999994,41.9950000000000,103.872000000000;0.0509999999999987,52.3980000000000,103.872000000000;0.0599999999999988,56.4680000000000,103.779000000000]\n\n%create racetrack trajectory\n\nLength=Rl/1000; %mm\nWidth=Rw/1000; %mm\n%turns radius = width/2\nAngle=[];\nfor i=0:20\n    Angle=[Angle;i*pi/20];\nend\n\nX=Width/2*sin(Angle)+Length/2\nY=-Width/2*cos(Angle)\n\nX2=-Width/2*sin(Angle)-Length/2\nY2=Width/2*cos(Angle)\n\nXtraj=[X;X2;X(1)]\nYtraj=[Y;Y2;Y(1)]\nZtraj=zeros(length(Xtraj),1)\nTraj=[Xtraj,Ytraj,Ztraj]\n\n\n[m,n]=size(Traj)\n\nVelocity=zeros(m,1)+2000;\nxoffsetVect=zeros(m,1)+xoffset;\nyoffsetVect=zeros(m,1)+yoffset;\nzoffsetVect=zeros(m,1)+zoffset;\n\n\n%TrajectoryOut=[(Traj(:,1).*xscale) +xoffset,(Traj(:,2).*yscale) +yoffset,(Traj(:,3).*zscale) +zoffset, Velocity]\nTrajectoryOut=[xscale.*Traj(:,1)+xoffsetVect,yscale.*Traj(:,2)+yoffsetVect,zscale.*Traj(:,3)+zoffsetVect, Velocity]\n\nFirstPoint=TrajectoryOut(1,:)\nTrajectoryOut=[TrajectoryOut]%;FirstPoint]\n%Test=TrajectoryOut(:,3)"("time"=w142, "xscale"=w138, "yscale"=w134, "zscale"=w133, "zoffset"=w137, "yoffset"=w136, "xoffset"=w135, "Rw"="Ractrack width [mm]", "Rl"="Racetrack length [mm]") -> ("TrajectoryOut"=w141:dbl[][])  [unwired: 1 in, 1 out]
              }
              frame "Circular" {
                n36 = mathscript code="%////////////////////////////////////////////////////////////////////\n%Calculate the coordinates of the points on a circle that will define the\n%trajectory\n%////////////////////////////////////////////////////////////////////\nXCircle=[];\nYCircle=[];\nZCircle=[];\nVelocity=[];\nCircleRadius=0.03;\nAngleCircle=0;\ni=1;\nwhile true\n    XCircle(i,1)=CircleRadius.*cos(AngleCircle);\n    YCircle(i,1)=CircleRadius.*sin(AngleCircle);\n    ZCircle(i,1)=0;\n    Velocity(i,1)=100; %m/s\n    AngleCircle=AngleCircle+0.05;\n    i=i+1\n    if AngleCircle>2*pi\n        break\n    end\nend\n%////////////////////////////////////////////////////////////////////\n\n%/////////////////////////////////////////////////////////////////\n%Calculate rotation matrix\nAngleXTrajectory=0;\nif Traj_R\nAngleYTrajectory=0.1.*time./1000;\nelse\nAngleYTrajectory=0.*time./1000;\nend\nRotationMatrixX=[1 0 0;0 cos(-AngleXTrajectory) -sin(-AngleXTrajectory);0 sin(-AngleXTrajectory) cos(-AngleXTrajectory)];\nRotationMatrixY=[cos(-AngleYTrajectory) 0 sin(-AngleYTrajectory);0 1 0 ; -sin(-AngleYTrajectory) 0 cos(-AngleYTrajectory)];\nRotationMatrix=RotationMatrixX*RotationMatrixY;\n\n%Make the rotation\nTrajectoryTemp=[];\n\nfor k=1:length(XCircle)\n \n   TrajectoryTemp(:,k)=RotationMatrix*[XCircle(k);YCircle(k);ZCircle(k)];\nend\n%TrajectoryOut=TrajectoryOut';\nTrajectoryTemp=TrajectoryTemp'\n\nTrajectoryOut=[ TrajectoryTemp , Velocity]"("time"=w668, "Traj_R"="Traj_Rotate") -> ("TrajectoryOut"=w666:dbl[][])  [unwired: 1 in, 1 out]
              }
              frame "Tube" {
                n37 = mathscript code="%////////////////////////////////////////////////////////////////////\n%Calculate the coordinates of the points on a circle that will define the\n%trajectory\n%////////////////////////////////////////////////////////////////////\n\n%Traj=0.001.*[-38.4570000000000,-39.0170000000000,12.5100000000000;-38.2850000000000,-37,18.8770000000000;-38.1630000000000,-35.5690000000000,23.3970000000000;-37.7350000000000,-34.4470000000000,26.9420000000000;-36.6090000000000,-33.9460000000000,28.5310000000000;-34.3690000000000,-33.5680000000000,29.7370000000000;-16.1370000000000,-33.4640000000000,29.9390000000000;-1.67200000000000,-25.2920000000000,29.9840000000000;1.98000000000000,-10.9570000000000,30;1.15900000000001,-4.81300000000000,31.9230000000000;0.822999999999993,-2.30400000000000,34.2870000000000;0.587000000000003,-0.536000000000001,37.5840000000000;0.509000000000000,0.0510000000000019,43.2310000000000;0.509000000000000,0.0510000000000019,53.5860000000000;0.0510000000000020,-0.509000000000000,64.1770000000000;0.0510000000000020,-0.509000000000000,79.3610000000000;0.0510000000000020,-0.509000000000000,93.5850000000000;0.0510000000000020,-0.432000000000002,97.4400000000000;0.0510000000000019,0.225999999999999,99.6090000000000;0.0510000000000018,1.68800000000000,101.676000000000;0.0510000000000016,5.40300000000001,103.720000000000;0.0510000000000005,24.2510000000000,103.872000000000;0.0509999999999994,41.9950000000000,103.872000000000;0.0509999999999987,52.3980000000000,103.872000000000;0.0599999999999988,56.4680000000000,103.779000000000;0.0799999999999946,59.5390000000000,102.836000000000;0.106999999999995,63.7900000000000,98.8510000000000;0.114000000000000,65.0030000000000,95.4370000000000;-17.2200000000000,65,94.3520000000000;-13.5000000000000,65,84;-24.5000000000000,65,71.4100000000000;-24.5000000000000,65,59.5060000000000;-24.5000000000000,65,46.0100000000000;-24.4530000000000,63.5720000000000,38.8830000000000;-24.3300000000000,59.7820000000000,33.8970000000000;-24.2250000000000,56.5810000000000,31.7900000000000;-24.1290000000000,53.6370000000000,30.7170000000000;-24.1060000000000,50.4100000000000,30.1660000000000;-24.7430000000000,47.2760000000000,29.3580000000000;-26.0920000000000,44.7010000000000,27.7300000000000;-29.3070000000000,42.4960000000000,23.9310000000000;-36.7150000000000,39.4140000000000,15.2170000000000;-39.0170000000000,38.4570000000000,12.5100000000000]\n%Traj=0.001.*[-38.4570000000000,-39.0170000000000,12.5100000000000;-38.2850000000000,-37,18.8770000000000;-38.1630000000000,-35.5690000000000,23.3970000000000;-37.7350000000000,-34.4470000000000,26.9420000000000;-36.6090000000000,-33.9460000000000,28.5310000000000;-34.3690000000000,-33.5680000000000,29.7370000000000;-16.1370000000000,-33.4640000000000,29.9390000000000;-1.67200000000000,-25.2920000000000,29.9840000000000;1.98000000000000,-10.9570000000000,30;1.15900000000001,-4.81300000000000,31.9230000000000;0.822999999999993,-2.30400000000000,34.2870000000000;0.587000000000003,-0.536000000000001,37.5840000000000;0.509000000000000,0.0510000000000019,43.2310000000000;0.509000000000000,0.0510000000000019,53.5860000000000;0.0510000000000020,-0.509000000000000,64.1770000000000;0.0510000000000020,-0.509000000000000,79.3610000000000;0.0510000000000020,-0.509000000000000,93.5850000000000;0.0510000000000020,-0.432000000000002,97.4400000000000;0.0510000000000019,0.225999999999999,99.6090000000000;0.0510000000000018,1.68800000000000,101.676000000000;0.0510000000000016,5.40300000000001,103.720000000000;0.0510000000000005,24.2510000000000,103.872000000000;0.0509999999999994,41.9950000000000,103.872000000000;0.0509999999999987,52.3980000000000,103.872000000000;0.0599999999999988,56.4680000000000,103.779000000000]\n\n%create racetrack trajectory\n\n%Traj=0.001*[-21,5.50000000000000,-18.3500000000000;-21,20.5000000000000,-18.5000000000000;-21,48,-18.5000000000000;-21,51,-19.1270000000000;-21,53.3000000000000,-20.6970000000000;-21,55.1840000000000,-23.8470000000000;-21,55.5000000000000,-28.5000000000000;-21,55.5000000000000,-48.5000000000000;-21,55.5000000000000,-68.5100000000000;-21,53.3000000000000,-73.8200000000000;-21,48,-76.0170000000000;-21,35.5960000000000,-76.0170000000000;-21,29.5900000000000,-76.0170000000000;-21,23.1920000000000,-76.0170000000000;-23.1970000000000,17.6970000000000,-76.0170000000000;-28.5000000000000,15.5000000000000,-76.0170000000000;-34.9500000000000,15.5000000000000,-76.0170000000000;-65.0500000000000,15.5000000000000,-76.0170000000000;-68.4300000000000,15.5000000000000,-76.0170000000000;-73.7300000000000,17.6900000000000,-76.0170000000000;-75.8600000000000,22.0340000000000,-76.0170000000000;-75.8600000000000,27.2700000000000,-76.0170000000000;-75.9300000000000,40.7900000000000,-76.0170000000000;-75.9300000000000,56.5400000000000,-76.0170000000000;-75.9300000000000,62.2900000000000,-76.0170000000000;-75.9300000000000,76.2600000000000,-76.0170000000000;-75.9300000000000,77.3300000000000,-75.5700000000000;-75.9300000000000,77.7600000000000,-74.5170000000000;-75.9300000000000,77.7600000000000,-70.7200000000000;-75.9300000000000,77.7600000000000,-60.2600000000000;-75.9300000000000,77.7600000000000,-21.3790000000000]\nTraj=0.001*[-21,5.50000000000000,-18.3500000000000;-21,20.5000000000000,-18.5000000000000;-21,48,-18.5000000000000;-21,51,-19.1270000000000;-21,53.3000000000000,-20.6970000000000;-21,55.1840000000000,-23.8470000000000;-21,55.5000000000000,-28.5000000000000;-21,55.5000000000000,-48.5000000000000;-21,55.5000000000000,-68.5100000000000;-21,53.3000000000000,-73.8200000000000;-21,48,-76.0170000000000;-21,35.5960000000000,-76.0170000000000;-21,29.5900000000000,-76.0170000000000;-21,23.1920000000000,-76.0170000000000;-23.1970000000000,17.6970000000000,-76.0170000000000;-28.5000000000000,15.5000000000000,-76.0170000000000;-34.9500000000000,15.5000000000000,-76.0170000000000;-65.0500000000000,15.5000000000000,-76.0170000000000;-68.4300000000000,15.5000000000000,-76.0170000000000;-73.7300000000000,17.6900000000000,-76.0170000000000;-75.8600000000000,22.0340000000000,-76.0170000000000;-75.8600000000000,27.2700000000000,-76.0170000000000;-75.9300000000000,40.7900000000000,-76.0170000000000;-75.9300000000000,56.5400000000000,-76.0170000000000;-75.9300000000000,62.2900000000000,-76.0170000000000;-75.9300000000000,76.7600000000000,-76.0170000000000;-75.9300000000000,77.7600000000000,-75.5700000000000;-75.9300000000000,77.7600000000000,-74.5170000000000;-75.9300000000000,77.7600000000000,-70.7200000000000;-75.9300000000000,77.7600000000000,-60.2600000000000;-75.9300000000000,77.7600000000000,-21.3790000000000]\nTraj=[-0.0210000000000000,0.00550000000000000,-0.0183500000000000;-0.0210000000000000,0.0205000000000000,-0.0185000000000000;-0.0210000000000000,0.0480000000000000,-0.0185000000000000;-0.0210000000000000,0.0510000000000000,-0.0191270000000000;-0.0210000000000000,0.0533000000000000,-0.0206970000000000;-0.0210000000000000,0.0551840000000000,-0.0238470000000000;-0.0210000000000000,0.0555000000000000,-0.0285000000000000;-0.0210000000000000,0.0555000000000000,-0.0485000000000000;-0.0210000000000000,0.0555000000000000,-0.0685100000000000;-0.0210000000000000,0.0533000000000000,-0.0738200000000000;-0.0210000000000000,0.0480000000000000,-0.0760170000000000;-0.0210000000000000,0.0355960000000000,-0.0760170000000000;-0.0210000000000000,0.0295900000000000,-0.0760170000000000;-0.0210000000000000,0.0231920000000000,-0.0760170000000000;-0.0231970000000000,0.0176970000000000,-0.0760170000000000;-0.0285000000000000,0.0155000000000000,-0.0760170000000000;-0.0349500000000000,0.0155000000000000,-0.0760170000000000;-0.0650500000000000,0.0155000000000000,-0.0760170000000000;-0.0737300000000000,0.0176900000000000,-0.0760170000000000;-0.0758600000000000,0.0220340000000000,-0.0760170000000000;-0.0758600000000000,0.0272700000000000,-0.0760170000000000;-0.0759300000000000,0.0407900000000000,-0.0760170000000000;-0.0759300000000000,0.0565400000000000,-0.0760170000000000;-0.0759300000000000,0.0622900000000000,-0.0760170000000000;-0.0759300000000000,0.0767600000000000,-0.0760170000000000;-0.0759300000000000,0.0777600000000000,-0.0755700000000000;-0.0759300000000000,0.0777600000000000,-0.0745170000000000;-0.0759300000000000,0.0777600000000000,-0.0707200000000000;-0.0759300000000000,0.0777600000000000,-0.0602600000000000;-0.0759300000000000,0.0777600000000000,-0.0213790000000000]\n\n\n\n[m,n]=size(Traj)\n\nVelocity=zeros(m,1)+2000;\nxoffsetVect=zeros(m,1)+xoffset;\nyoffsetVect=zeros(m,1)+yoffset;\nzoffsetVect=zeros(m,1)+zoffset;\n\n\n%TrajectoryOut=[(Traj(:,1).*xscale) +xoffset,(Traj(:,2).*yscale) +yoffset,(Traj(:,3).*zscale) +zoffset, Velocity]\n\nTrajectoryOut=[xscale.*Traj(:,1)+xoffsetVect,-yscale.*Traj(:,3)+yoffsetVect,zscale.*Traj(:,2)+zoffsetVect, -Velocity]\n\n%TrajectoryOut=[xscale.*Traj(:,1)+xoffsetVect,-yscale.*Traj(:,3)+yoffsetVect,zscale.*Traj(:,2)+zoffsetVect, Velocity]\n\n\nFirstPoint=TrajectoryOut(1,:)\nTrajectoryOut=[TrajectoryOut]%;FirstPoint]\n%Test=TrajectoryOut(:,3)"("xscale"=w1170, "yscale"=w1169, "zscale"=w1168, "zoffset"=w1171, "yoffset"=w1173, "xoffset"=w1172) -> ("TrajectoryOut"=w1174:dbl[][])  [unwired: 1 in, 1 out]
              }
            }
          }
          frame #2 {
            # "Analytical Model"
            # "Trajectory controller"
            n38 = global read "Global 2.vi" "Measure"() -> (w1444:bool)
            n39 = global read "Global 2.vi" "X"() -> (w1458:dbl)
            n40 = global read "Global 2.vi" "Y"() -> (w1457:dbl)
            n41 = global read "Global 2.vi" "Z"() -> (w1451:dbl)
            n42 = call "TrajectoryController.vi"("X"=w1458, "Y"=w1457, "Z"=w1451, "Trajectory"=w1456) -> ("error"=w1443:cdb, "XHD"=w1454:dbl[], "AccelerationOverVsquare"=w1449:dbl[], "Yclosest"=w1450:dbl, "Xclosest"=w1445:dbl, "Zclosest"=w1452:dbl, "ZHD"=w1455:dbl[], "YHD"=w1453:dbl[], "OptimumVelocity"=w1436:dbl[])  [unwired: 3 in]
            "Array" <- w1436
            n43 = mathscript code="XCircleBot=[];\nYCircleBot=[];\nZCircleBot = [];\nCircleRadius=0.002;\nAngleCircle=0;\ni=0\nwhile true\n     i=i+1\n    XCircleBot(i)=CircleRadius.*cos(AngleCircle);\n    YCircleBot(i)=CircleRadius.*sin(AngleCircle);\n    %ZCircleBot(i) = 0;\n    AngleCircle=AngleCircle+0.5;\n\n    if AngleCircle>2*pi\n        break\n    end\nend\nXCircleBotOut=XCircleBot+XPos;\nYCircleBotOut=YCircleBot+YPos;\nZCircleBotOut=YCircleBot+ZPos;\n\nXCircleClosestOut=XCircleBot+Xclosest;\nYCircleClosestOut=YCircleBot+Yclosest;\nZCircleClosestOut=YCircleBot+Zclosest;\n\nError=sqrt(((XPos-Xclosest).^2)+((YPos-Yclosest).^2)+((ZPos-Zclosest).^2))"("XPos"=w1458, "YPos"=w1457, "Xclosest"=w1445, "Yclosest"=w1450, "ZPos"=w1451, "Zclosest"=w1452) -> ("XCircleBotOut"=w1467:dbl[], "YCircleBotOut"=w1470:dbl[], "XCircleClosestOut"=w1465:dbl[], "YCircleClosestOut"=w1469:dbl[], "ZCircleClosestOut"=w1466:dbl[], "ZCircleBotOut"=w1468:dbl[])  [unwired: 1 in, 2 out]
            n44 = case shown="False" w1444 {
              tunnel: [0.0 w1476] -> _
              tunnel: w1443 -> [_ w1476]
              frame False {
              }
              frame True {
              }
            }
            n45 = Bundle("XHD"=w1454, "ZHD"=w1455) -> (w1463:cluster{"XHD":dbl[], "ZHD":dbl[]})  [unwired: 1 in]
            n46 = Bundle("XHD"=w1454, "YHD"=w1453) -> (w1460:cluster{"XHD":dbl[], "YHD":dbl[]})  [unwired: 1 in]
            n47 = Bundle("XCircleClosestOut"=w1465, "ZCircleClosestOut"=w1466) -> (w1462:T5)  [unwired: 1 in]
            n48 = Bundle("XCircleBotOut"=w1467, "ZCircleBotOut"=w1468) -> (w1464:T6)  [unwired: 1 in]
            n49 = Bundle("XCircleClosestOut"=w1465, "YCircleClosestOut"=w1469) -> (w1461:T7)  [unwired: 1 in]
            n50 = Bundle("XCircleBotOut"=w1467, "YCircleBotOut"=w1470) -> (w1459:T8)  [unwired: 1 in]
            n51 = case shown="False" "Reverse" {
              tunnel: [1 -1] -> w1441
              tunnel: [w1471 w1473] -> w1439
              tunnel: "CD" -> [w1471 _]
              tunnel: "CDB" -> [_ w1473]
              frame False {
              }
              frame True {
              }
            }
            n52 = mathscript code="%/////////////////////////////////////////////////////////////////\n%Fluid mechanics analytical model\n%///////////////////////////////////////////////////////\nBotDiameter=0.005; %[m]\n%CD=0.002; %drag coeficient \nRho=1000; %[Kg/m3]\nVopt = norm(OptimumVelocity)\nFd=CD.*Rho.*Vopt.*pi.*BotDiameter.*BotDiameter/4;\nFdVect=Fd.*OptimumVelocity./norm(OptimumVelocity);\n\n%Calculate the weight of the robot\nmass=0.0001; %[Kg]\nWeight=[0,0,-mass.*9.81]\n\n%Calculate the centripedal force\nif CFCactive\nFCF=Acceleration.*KCF\nelse\nFCF=[0,0,0]\nend"("OptimumVelocity"=w1436, "Acceleration"=w1449, "KCF"="KCentripedal force", "CFCactive"="Centripedal force compensation", "CD"=w1439) -> ("FdVect"=w1442:dbl[], "FCF"=w1447:dbl[])  [unwired: 1 in, 1 out]
            "?" <- "Centripedal force compensation"
            "Boolean" <- "Reverse"
          }
          frame #3 {
            # "DeltaT [s]"
            # "deltaT [ms]"
            # "Z closest"
            # "Y closest"
            # "X closest"
            # "PID controller"
            # "z"
            # "y"
            # "x"
            n53 = case shown="True" "Reset Integral" {
              tunnel: w1981 -> [w2001 _]
              tunnel: [w2001 w2002] -> w1979
              frame False {
              }
              frame True {
                n54 = mathscript code="I=[0.0;0.0;0.0]"() -> ("I"=w2002:dbl[])  [unwired: 1 in, 1 out]
              }
            }
            n55 = Divide(x=w1985, y=1000.0) -> (x/y=w1983:dbl)
            n56 = case shown="True" w1978 {
              tunnel: [w1997 w1999] -> w1977
              tunnel: "Ki" -> [w1997 _]
              tunnel: [w1996 w2000] -> w1975
              tunnel: "Kp" -> [w1996 _]
              tunnel: [w1995 w1998] -> w1973
              tunnel: "Kd" -> [w1995 _]
              tunnel: "KpB" -> [_ w2000]
              tunnel: "KiB" -> [_ w1999]
              tunnel: "KdB" -> [_ w1998]
              frame False {
              }
              frame True {
              }
            }
            n57 = call "PID.vi"("Z"=w1989, "Xclosest"=w1986, "ErrorIn"=w1992, "Yclosest"=w1987, "Zclosest"=w1988, "Kp"=w1975, "Ki"=w1977, "IntegralIn"=w1979, "Y"=w1990, "Kd"=w1973, "X"=w1991, "deltaT"=w1983) -> ("FPID"=w1982:dbl[], "IntegralOut"=w1994:dbl[], "ErrorOut"=w1993:dbl[])  [unwired: 13 in]
          }
          frame #4 {
            # "Centripedal force"
            # "Drag Force"
            # "FPId"
            # "Sum all the components of the force"
            n58 = mathscript code="G=9.81; %[m/s^2]\nW=[0;0;Mass.*G]"("Mass"="Robot Mass [Kg]") -> ("W"=w2067:dbl[])  [unwired: 1 in, 1 out]
            n59 = case shown="True" w2035 {
              tunnel: [w2069 w2070] -> w2038
              tunnel: "Thrust coefficient [N.s/rad]" -> [w2069 _]
              tunnel: "ThrustCoefB" -> [_ w2070]
              frame False {
              }
              frame True {
              }
            }
            n60 = mathscript code="FPID=Direction*FPID\nW=Direction*W\nFr=[FPID(1)+DragF(1)+W(1)+FCF(1);FPID(2)+DragF(2)+W(2)+FCF(1);FPID(3)+DragF(3)+W(3)+FCF(3)]\nDirectionSetpoint=Fr./norm(Fr);\nF = norm(Fr)\n%Calculate vectors to plot the direction of the froce to be applied\nScaleFactor=0.05;\n\nXPlot=[X,X+ScaleFactor.*DirectionSetpoint(1)]\nYPlot=[Y,Y+ScaleFactor.*DirectionSetpoint(2)]\nZPlot=[Z,Z+ScaleFactor.*DirectionSetpoint(3)]\n\nOmega=norm(Fr)./TC;\n\nif Direction==1\nif Omega >70*2*pi\nOmega = 70*2*pi\nend\n\n\nif Omega <-70*2*pi\nOmega = -70*2*pi\nend\nend\nif Direction==-1\nif Omega >75*2*pi\nOmega = 75*2*pi\nend\n\n\nif Omega <-75*2*pi\nOmega = -75*2*pi\nend\nend\n%if abs(Omega) > 160\n%Omega = -160\n%end\n\n%if abs(Omega) <130\n%Omega = -130\n%end\n\nif abs(Omega-Omega_in)>Omega_Max\nOmega_out = Omega + sign(Omega - Omega_in)\nelse\nOmega_out = Omega\nend\n\n%Calculate vectors to plot the direction of the froce to be applied\nScaleFactor=0.001;\n\nXaccPlot=[X,X+ScaleFactor.*AccelerationOverVsquare(1)]\nYaccPlot=[Y,Y+ScaleFactor.*AccelerationOverVsquare(2)]\nZaccPlot=[Z,Z+ScaleFactor.*AccelerationOverVsquare(3)]\n\n%Calculate the magnetization of the magnet\nM=1.06E-3; %magnetic moment\nMagneticMomentVector=M*DirectionSetpoint;\nmx=MagneticMomentVector(1)\nmy=MagneticMomentVector(2)\nmz=MagneticMomentVector(3)"("FPID"=w2066, "DragF"=w2065, "W"=w2067, "X"=w2063, "Y"=w2062, "Z"=w2061, "TC"=w2038, "Omega_in"=w2057, "Omega_Max"="Omega_Max_change", "AccelerationOverVsquare"=w2055, "FCF"=w2043, "Direction"=w2039) -> ("DirectionSetpoint"=w2064:dbl[], "XPlot"=w2053:dbl[], "YPlot"=w2052:dbl[], "ZPlot"=w2048:dbl[], "Omega_out"=w2058:dbl, "XaccPlot"=w2047:dbl[], "YaccPlot"=w2046:dbl[], "ZaccPlot"=w2045:dbl[], "mx"=w2042:dbl, "my"=w2041:dbl, "mz"=w2040:dbl)  [unwired: 1 in, 2 out]
            n61 = case shown="False" "?" {
              tunnel: [w2073 w2075] -> w2054
              tunnel: w2053 -> [_ w2075]
              tunnel: w2052 -> [_ w2076]
              tunnel: [w2072 w2076] -> w2051
              tunnel: [w2073 w2075] -> w2050
              tunnel: [w2071 w2074] -> w2049
              tunnel: w2048 -> [_ w2074]
              tunnel: w2047 -> [w2073 _]
              tunnel: w2046 -> [w2072 _]
              tunnel: w2045 -> [w2071 _]
              frame False {
              }
              frame True {
              }
            }
            n62 = Bundle("XPlot"=w2050, "ZPlot"=w2049) -> (w2059:cluster{"XPlot":dbl[], "ZPlot":dbl[]})  [unwired: 1 in]
            n63 = Bundle("XPlot"=w2054, "YPlot"=w2051) -> (w2060:cluster{"XPlot":dbl[], "YPlot":dbl[]})  [unwired: 1 in]
          }
          frame #5 {
            n64 = mathscript code="%/////////////////////////////////////////////////////////////////////////////////////////\n%Calculate the two rotation angles\n%/////////////////////////////////////////////////////////////////////////////////////////\n%Find the values of the angles of direction Setpoint\n%AngleY=asin(DirectionSetpoint(1))\n%AngleX=acos(DirectionSetpoint(3)./cos(AngleY))\n\n%AngleX=sign(DirectionSetpoint(2)).*AngleX;\n%AngleY=-1.*AngleY;\n\n\n%AngleY=asin(DirectionSetpoint(1))\n%AngleX=acos(DirectionSetpoint(3)./cos(AngleY))\n\n%AngleX=sign(DirectionSetpoint(2)).*AngleX;\n%AngleY=-1.*AngleY;\n %AngleX =-atan2(DirectionSetpoint(2),sqrt(DirectionSetpoint(3)^2+DirectionSetpoint(1)^2));\n %AngleY =-sign(DirectionSetpoint(1)).*( atan2(DirectionSetpoint(1),DirectionSetpoint(3)));\n\nAngleY=asin(DirectionSetpoint(1))\nAngleX=acos(DirectionSetpoint(3)./cos(AngleY))\n\nAngleX=-sign(DirectionSetpoint(2)).*AngleX;\n%AngleY=1.*AngleY;\n\n%AngleX=-atan2(DirectionSetpoint(2),sqrt(DirectionSetpoint(3)^2+DirectionSetpoint(1)^2));\n%AngleY=atan2(DirectionSetpoint(1),DirectionSetpoint(3))\n\n\n%Detect a completed rotation and modify PreviousAngleX acordingely\nif AngleX-PreviousAngleX>pi\nPreviousAngleX=PreviousAngleX+2.*pi\nend\nif AngleX-PreviousAngleX<-pi\nPreviousAngleX=PreviousAngleX-2.*pi\nend\nif AngleY-PreviousAngleY>pi\nPreviousAngleX=PreviousAngleX+2.*pi\nend\nif AngleY-PreviousAngleY<-pi\nPreviousAngleY=PreviousAngleY-2.*pi\nend\n\nVariationSpeedX=(AngleX-PreviousAngleX)./(DeltaT./1000)\nVariationSpeedY=(AngleY-PreviousAngleY)./(DeltaT./1000)\n\nif abs(VariationSpeedX)>MaxChangeRate\nAngleX=PreviousAngleX+MaxChangeRate.*(DeltaT./1000).*sign(VariationSpeedX)\nend\n\nif abs(VariationSpeedY)>MaxChangeRate\nAngleY=PreviousAngleY+MaxChangeRate.*(DeltaT./1000).*sign(VariationSpeedY)\nend\n\n\n\nif ForceVertical\nAngleX=0;\nAngleY=0;\nend"("DirectionSetpoint"=w2897, "ForceVertical"="Force Vertical", "PreviousAngleX"=w2893, "PreviousAngleY"=w2892, "MaxChangeRate"="Max Orientation change rate [rad/s]", "DeltaT"=w2895) -> ("AngleX"=w2891:cdb, "AngleY"=w2890:cdb)  [unwired: 1 in, 1 out]
          }
          frame #6 {
            # "dBv/dt"
            # "dBu/dt"
            # "Electromagnetic calculation"
            n65 = case shown="False" "Rotational speed" {
              tunnel: w3312 -> [_ w3346]
              tunnel: [w3345 w3346] -> w3308
              frame False {
                n66 = Multiply(x=6.283, y="Rot [Hz]") -> (x*y=w3345:dbl)
              }
              frame True {
              }
            }
            n67 = Divide(x=w3330, y=1000.0) -> (x/y=w3332:dbl)
            n68 = Multiply(x=w3308, y=w3307) -> (x*y=w3303:dbl)
            n69 = Divide(x=w3303, y=6.283) -> (x/y=→"Rotation speed [Hz]":dbl)
            n70 = call "RotatingFieldCalculation_uvw.vi"("Time Step (ms)"=w3311, "Flux density magnitude (T)"=w3332, "Previous Field Angle (rad)"=w3341, "Omega (rad/s)"=w3303) -> ("Bv (T)"=w3304:sgl, "Bu (T)"=w3302:sgl, "New Field Angle (rad)"=w3342:sgl)  [unwired: 5 in]
            n71 = call "FieldPlaneRotation.vi"("Bv (T)"=w3304, "Bu (T)"=w3302, "AlfaY (rad)"=w3298, "AlfaX (rad)"=w3299) -> ("Bz (T)"=w3338:dbl, "By (T)"=w3339:dbl, "Bx (T)"=w3340:dbl)  [unwired: 5 in]
            n72 = Multiply(x=w3303, y=-1.0) -> (x*y=w3305:dbl)
            n73 = Multiply(x=w3305, y=w3304) -> (x*y=w3301:dbl)
            n74 = Multiply(x=w3303, y=w3302) -> (x*y=w3300:dbl)
            n75 = shared-variable "NI-IC-3173-01BA58CC\\EtherCAT Master\\Device\\Mod3\\TC3"() -> (w3321:dbl)  [unwired: 1 in, 1 out]
            "X+" <- w3321
            "T4" <- w3321
            n76 = shared-variable "NI-IC-3173-01BA58CC\\EtherCAT Master\\Device\\Mod3\\TC4"() -> (w3322:dbl)  [unwired: 1 in, 1 out]
            "Y-" <- w3322
            "T5" <- w3322
            n77 = shared-variable "NI-IC-3173-01BA58CC\\EtherCAT Master\\Device\\Mod3\\TC5"() -> (w3323:dbl)  [unwired: 1 in, 1 out]
            "Y+" <- w3323
            "T6" <- w3323
            n78 = shared-variable "NI-IC-3173-01BA58CC\\EtherCAT Master\\Device\\Mod3\\TC2"() -> (w3320:dbl)  [unwired: 1 in, 1 out]
            "X-" <- w3320
            "T3" <- w3320
            n79 = shared-variable "NI-IC-3173-01BA58CC\\EtherCAT Master\\Device\\Mod3\\TC1"() -> (w3319:dbl)  [unwired: 1 in, 1 out]
            "Z+" <- w3319
            "T2" <- w3319
            n80 = shared-variable "NI-IC-3173-01BA58CC\\EtherCAT Master\\Device\\Mod3\\TC6"() -> (w3318:dbl)  [unwired: 1 in, 1 out]
            "Z-" <- w3318
            "T1" <- w3318
            n81 = call "FieldPlaneRotation.vi"("Bv (T)"=w3300, "Bu (T)"=w3301, "AlfaY (rad)"=w3298, "AlfaX (rad)"=w3299) -> ("Bz (T)"=w3295:dbl, "By (T)"=w3296:dbl, "Bx (T)"=w3297:dbl)  [unwired: 5 in]
            n82 = call "VoltageController.vi"("Y (m)"=w3316, "X (m)"=w3315, "dBzdt"=w3295, "Z (m)"=w3317, "dBxdt"=w3297, "Bx [T]"=w3340, "By [T]"=w3339, "Bz [T]"=w3338, "dBydt"=w3296) -> ("XN"=w3337:dbl, "XP"=w3294:dbl, "YN"=w3293:dbl, "YP"=w3336:dbl, "ZP"=w3334:dbl, "ZN"=w3335:dbl)  [unwired: 1 in]
            "v2" <- w3294
            "v1" <- w3293
            n83 = mathscript code="if T1 > TempSet || T2 > TempSet || T3 > TempSet || T4 > TempSet || T5 > TempSet || T6 > TempSet\nOverTemp=true\nelse\nOverTemp=false\nend\n\nif ~OverTemp && On_Off\nOn_Off_Out=true\nelse\nOn_Off_Out=false\nend"("T1"=w3318, "T2"=w3319, "T3"=w3320, "T4"=w3321, "T5"=w3322, "T6"=w3323, "On_Off"="On Off", "TempSet"="Max Temp[C]") -> ("On_Off_Out"=w3325:bool, "OverTemp"=→"OverTemp":bool)  [unwired: 1 in, 1 out]
            "On" <- w3325
            n84 = call "PowerSupplyControl.vi"("OnOff"=w3325, "Max Current (A)"=w3328, "Z-"=w3335, "X+"=w3294, "Z+"=w3334, "Y-"=w3293, "Y+"=w3336, "X-"=w3337) -> ("Saturating"=→"Current Saturation":bool, "Max Current"=w3329:dbl)  [unwired: 2 in]
            n85 = Divide(x=w3312, y=6.283) -> ()  [unwired: 1 out]
          }
        }
        "Max Current [A]" <- w114
        n86 = Bundle(w100, w99, w98, w91) -> (w102:T9)  [unwired: 1 in]
        n87 = Bundle(w93, w94, w95, w92) -> (w97:T10)  [unwired: 1 in]
        n88 = Cluster To Array(cluster=w102) -> (array=→"XZ View":cluster{"XPlot":dbl[], "ZPlot":dbl[]}[])
        n89 = Cluster To Array(cluster=w97) -> (array=→"XY View":cluster{"XPlot":dbl[], "YPlot":dbl[]}[])
        n90 = node-c288() -> ()  [unwired: 1 in, 1 out]
      }
      n91 = node-c288(w86) -> ()  [unwired: 1 out]
    }
  }
